vi "DRAW_Full_Trajectory_(offline).vi"(0 "Image In":T1, 5 "Animal coordinates and speed":T3, 7 "Mouse drawing parameters":T4, 9 "Size of the image (480x480)":T5={"Numeric Control"=480.0, "Numeric Control"=480.0}, 11 "Error In":errorcluster) -> (4 "Images out":T2, 15 "Error Out":errorcluster)   [LabVIEW 2018, in "Tracker.lvlib"]
uses:
  Tracker.lvlib
  <vilib>/vision/Image Controls.llb/IMAQ Image.ctl
  Controls/CTL_Mouse_Draw_Params.ctl
  Controls/CTL_Animal_Coordinates_and_Speed_(arr).ctl
  <vilib>/Utility/miscctls.llb/LVBoundsTypeDef.ctl
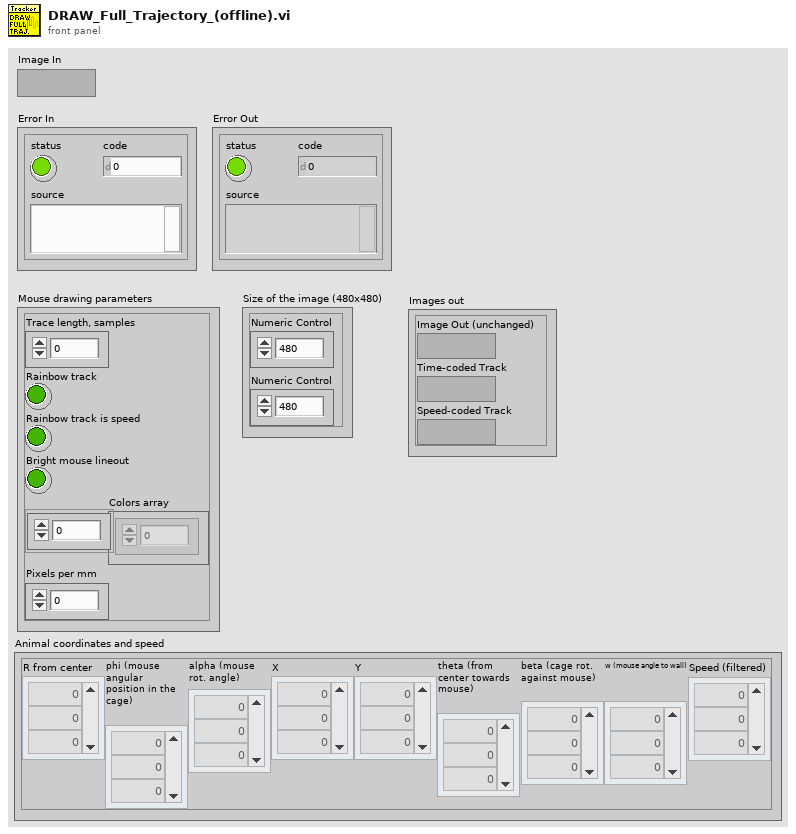
[diagram p1: front panel]
types:
  T1 = typedef "IMAQ Image.ctl" = refnum<image>
  T2 = cluster{"Image Out (unchanged)":T1, "Time-coded Track":T1, "Speed-coded Track":T1}
  T3 = typedef "Tracker.lvlib/CTL_Animal_Coordinates_and_Speed_(arr).ctl" = cluster{"R from center":dbl[], "phi (mouse angular position in the cage)":dbl[], "alpha (mouse rot. angle)":dbl[], "X":dbl[], "Y":dbl[], "theta (from center towards mouse)":dbl[], "beta (cage rot. against mouse)":dbl[], "w (mouse angle to wall)":dbl[], "Speed (filtered)":dbl[]}
  T4 = typedef "Tracker.lvlib/CTL_Mouse_Draw_Params.ctl" = cluster{"Trace length, samples":u16, "Rainbow track":bool, "Rainbow track is speed":bool, "Bright mouse lineout":bool, "Colors array":u32[], "Pixels per mm":dbl}
  T5 = cluster{"Numeric Control":dbl, "Numeric Control":dbl}
  T6 = typedef "LVBoundsTypeDef.ctl" = cluster{"Width":u32, "Height":u32}
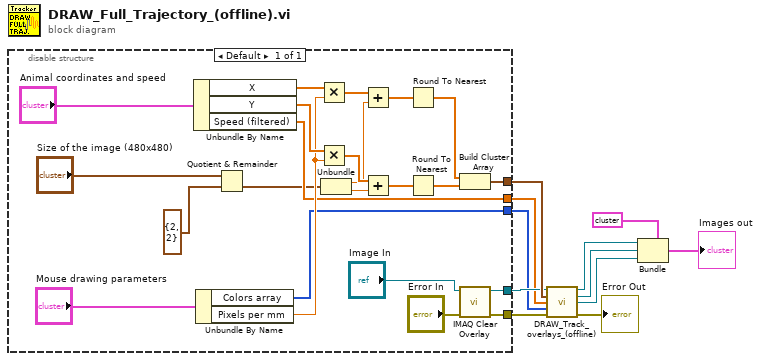
[diagram p0: block diagram]
diagram:
  n1 = disable-structure shown="Default" {
    disable-tunnel: [w27] -> w8
    disable-tunnel: [w17] -> w11
    disable-tunnel: [w15] -> w10
    disable-tunnel: [w14] -> w9
    disable-tunnel: [w12] -> w6
    frame Enabled {
      n2 = Unbundle By Name("Animal coordinates and speed") -> ("X"=w32:dbl[], "Y"=w31:dbl[], "Speed (filtered)"=w27:dbl[])
      n3 = Unbundle By Name("Mouse drawing parameters") -> ("Colors array"=w14:u32[], "Pixels per mm"=w29:dbl)
      n4 = Quotient & Remainder(x="Size of the image (480x480)", y=T6 {"Width"=2, "Height"=2}) -> (floor(x/y)=w24:cluster{dbl, dbl})  [unwired: 1 out]
      n5 = Multiply(x=w32, y=w29) -> (x*y=w34:dbl[])
      n6 = Multiply(x=w31, y=w29) -> (x*y=w33:dbl[])
      n7 = Unbundle(w24) -> (w21:dbl, w20:dbl)
      n8 = Add(x=w34, y=w21) -> (x+y=w23:dbl[])
      n9 = Add(x=w33, y=w20) -> (x+y=w22:dbl[])
      n10 = Round To Nearest(number=w23) -> (nearest integer value=w19:dbl[])
      n11 = Round To Nearest(number=w22) -> (nearest integer value=w18:dbl[])
      n12 = Build Cluster Array(w19, w18) -> (w17:cluster{dbl, dbl}[])
      n13 = call "IMAQ Clear Overlay"("error in (no error)"="Error In", "Image"="Image In") -> ("error out"=w12:errorcluster, "Image Out"=w15:T1)  [unwired: 8 in]
    }
  }
  n14 = call "DRAW_Track_overlays_(offline).vi"("Image In"=w10, "Full track array"=w11, "Speed array"=w8, "Colors array input"=w9, "Error In"=w6) -> ("Image Out (unchanged)"=w5:T1, "Time-coded Track"=w4:T1, "Speed-coded Track"=w3:T1, "Error Out"=→"Error Out":errorcluster)  [unwired: 7 in]
  n15 = Bundle(cluster=T2 {"Image Out (unchanged)"=refnum, "Time-coded Track"=refnum, "Speed-coded Track"=refnum} ("Images out"), "Image Out (unchanged)"=w5, "Time-coded Track"=w4, "Speed-coded Track"=w3) -> (→"Images out":T2)
